vi "preptempbuffers.vi"   [LabVIEW 2015]
types:
  T1 = typedef "LVRectTypeDef.ctl" = cluster{"Left":i16, "Top":i16, "Right":i16, "Bottom":i16}
  T2 = cluster{"Xpixels":i32, "Vxminref":dbl, "Vxmaxref":dbl, "P":dbl, "Ypixels":i32, "Vyminref":dbl, "Vymaxref":dbl, "srate":sgl, "sAOxy":i32, "timeout":dbl, "type":string, "date":string, "time":string, "Colormap":u16, "Drawing Mode":u16, "Scanning Mode":u16, "square pixels":bool, "square matrix":bool, "Xpixels Img":i32, "Vx-min Img":dbl, "VX-max Img":dbl, "Ypixels Img":i32, "Vy-min Img":dbl, "Vy-max Img ":dbl, "Angle Img":dbl, "autoshutter":bool, "finite":bool, "cont":bool, "wavdet":bool, "measpoints":i32, "avpp":i32, "bufferAO":i32, "bufferAI":i32, "starttick":u32, "waveform":path, "Vx-ref":dbl, "Vy-ref":dbl, "refreshrate":dbl, "refreshbuffer":i32, "tt_cycles":i32, "motorref":refnum<k7>, "mirrorswitch":refnum<k7>, "sample mode":i32, "maxbufferAI":i32, "srateAODO":sgl, "bin":sgl, "Pel":sgl, "Angle draw":dbl, "srate Img":sgl, "ROIimg_plotbounds":T1, "auto OD":bool, "ODfilt":u16, "aAI":i32[], "aCI":i32[], "aAO":u32[], "aDO":u32[], "refwfsize":dbl, "Lifetime":bool, "Vz-Img":dbl, "Vz-ref":dbl, "Vz-reset":dbl, "AIoverride":bool}
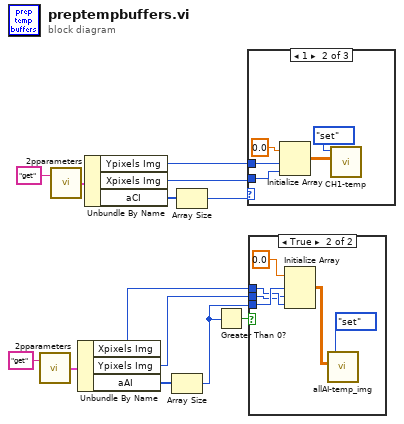
[diagram p0: block diagram]
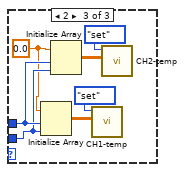
[diagram p4: hidden frame]
diagram:
  n1 = call "2pparameters.vi"("command"="get") -> ("params out"=w10:T2)  [unwired: 1 in]
  n2 = call "2pparameters.vi"("command"="get") -> ("params out"=w12:T2)  [unwired: 1 in]
  n3 = Unbundle By Name(w10) -> ("Xpixels Img"=w8:i32, "Ypixels Img"=w7:i32, "aAI"=w6:i32[])
  n4 = Unbundle By Name(w12) -> ("Ypixels Img"=w2:i32, "Xpixels Img"=w1:i32, "aCI"=w13:i32[])
  n5 = Array Size(array=w6) -> (size(s)=w4:i32)
  n6 = Array Size(array=w13) -> (size(s)=w3:i32)
  n7 = Greater Than 0?(x=w4) -> (x > 0?=w5:bool)
  n8 = case shown="1" w3 {
    tunnel: w2 -> [_ w15 w21]
    tunnel: w1 -> [_ w14 w20]
    frame 0, Default {
    }
    frame 1 {
      n9 = Initialize Array(sgl 0.0 ("element"), w15, w14) -> (w16:sgl[][])
      n10 = call "CH1-temp.vi"("array in"=w16, "command"=enum16{"get", "set", "clear", "add row"}."set") -> ()  [unwired: 2 in, 2 out]
    }
    frame 2 {
      w19 = sgl 0.0 ("element")
      n11 = Initialize Array(w19, w21, w20) -> (w24:sgl[][])
      n12 = Initialize Array(w19, w21, w20) -> (w23:sgl[][])
      n13 = call "CH1-temp.vi"("array in"=w24, "command"=enum16{"get", "set", "clear", "add row"}."set") -> ()  [unwired: 2 in, 2 out]
      n14 = call "CH2-temp.vi"("array in"=w23, "command"=enum16{"get", "set", "clear", "add row"}."set") -> ()  [unwired: 2 in, 2 out]
    }
  }
  n15 = case shown="True" w5 {
    tunnel: w8 -> [_ w27]
    tunnel: w7 -> [_ w26]
    tunnel: w4 -> [_ w28]
    frame False {
    }
    frame True {
      n16 = Initialize Array(sgl 0.0 ("element"), w28, w26, w27) -> (w31:sgl[][][])
      n17 = call "allAI-temp_img.vi"("array in"=w31, "command"=enum16{"get", "set", "clear", "append"}."set") -> ()  [unwired: 2 in, 2 out]
    }
  }
